vi "Page_AddProject.vi"(8 "error in (no error)":errorcluster, 11 "Configuration Paths in":T1) -> (0 "error out":errorcluster, 3 "Configuration Paths out":T1)   [LabVIEW 2010]
uses:
  Config cluster.ctl
panel:
  in  "Delete":bool
  in  "OK":bool
  in  "Selected Project Files":i32(listbox)
  in  "Configuration Files":i32(listbox)=-1
  in  "Cancel":bool
  in  "Add Proj":bool
  in  "Mode":enum16{"MIL", "HIL", "XiL"}(ring)
  # "1) Choose the type of test to be performed"
  # "2) Select the configuration files that will be used in the test(s)"
  # "Available Project Files"
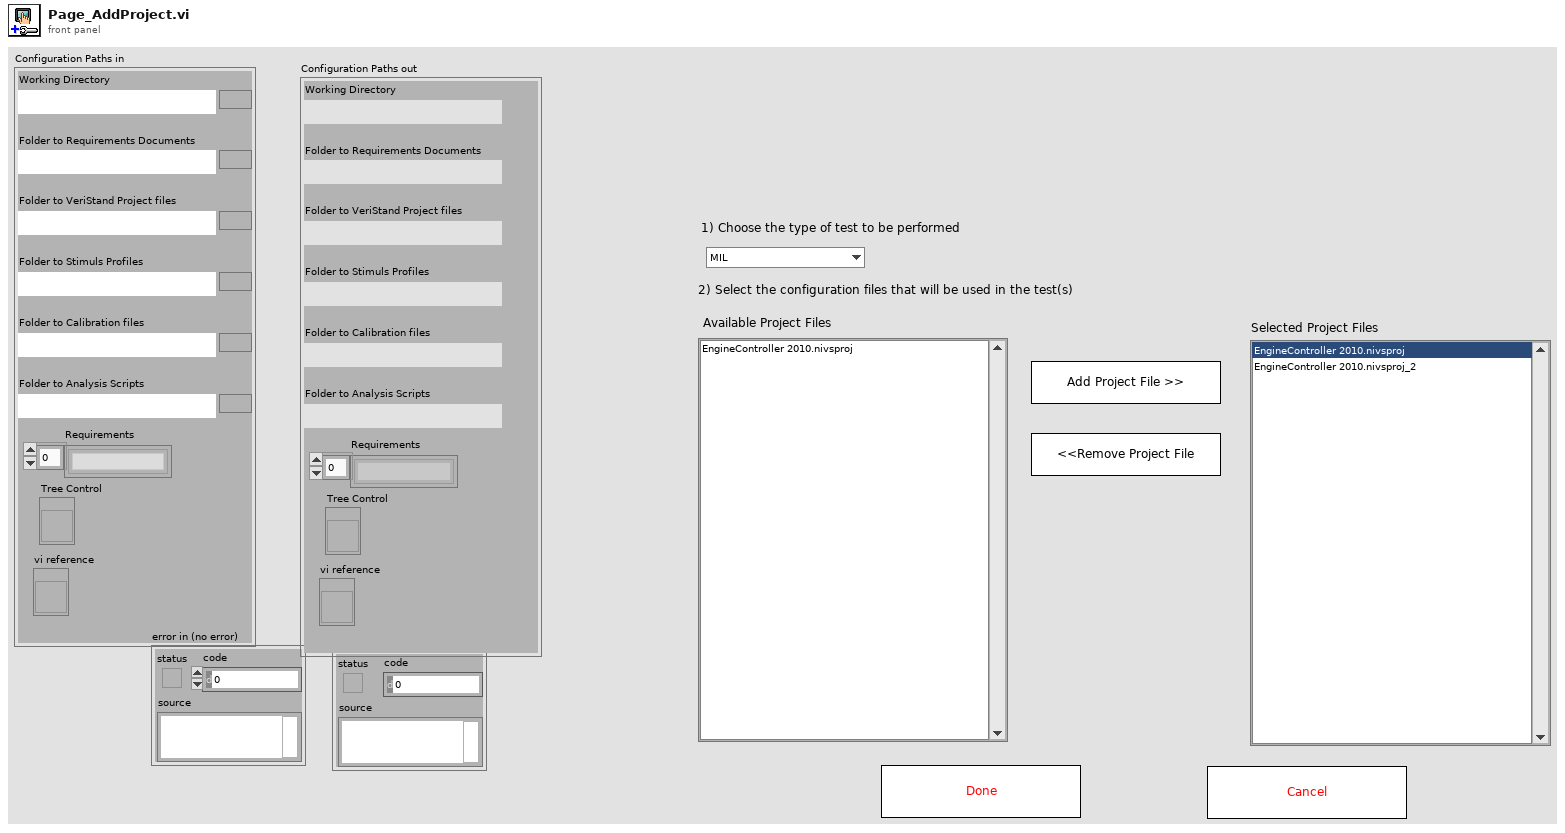
[diagram p1: front panel]
types:
  T1 = typedef "Config cluster.ctl" = cluster{"Working Directory":path, "Folder to Requirements Documents":path, "Folder to VeriStand Project files":path, "Folder to Stimuls Profiles":path, "Folder to Calibration files":path, "Folder to Analysis Scripts":path, "Requirements":string[], "Tree Control":refnum<vi>, "vi reference":refnum<vi>}
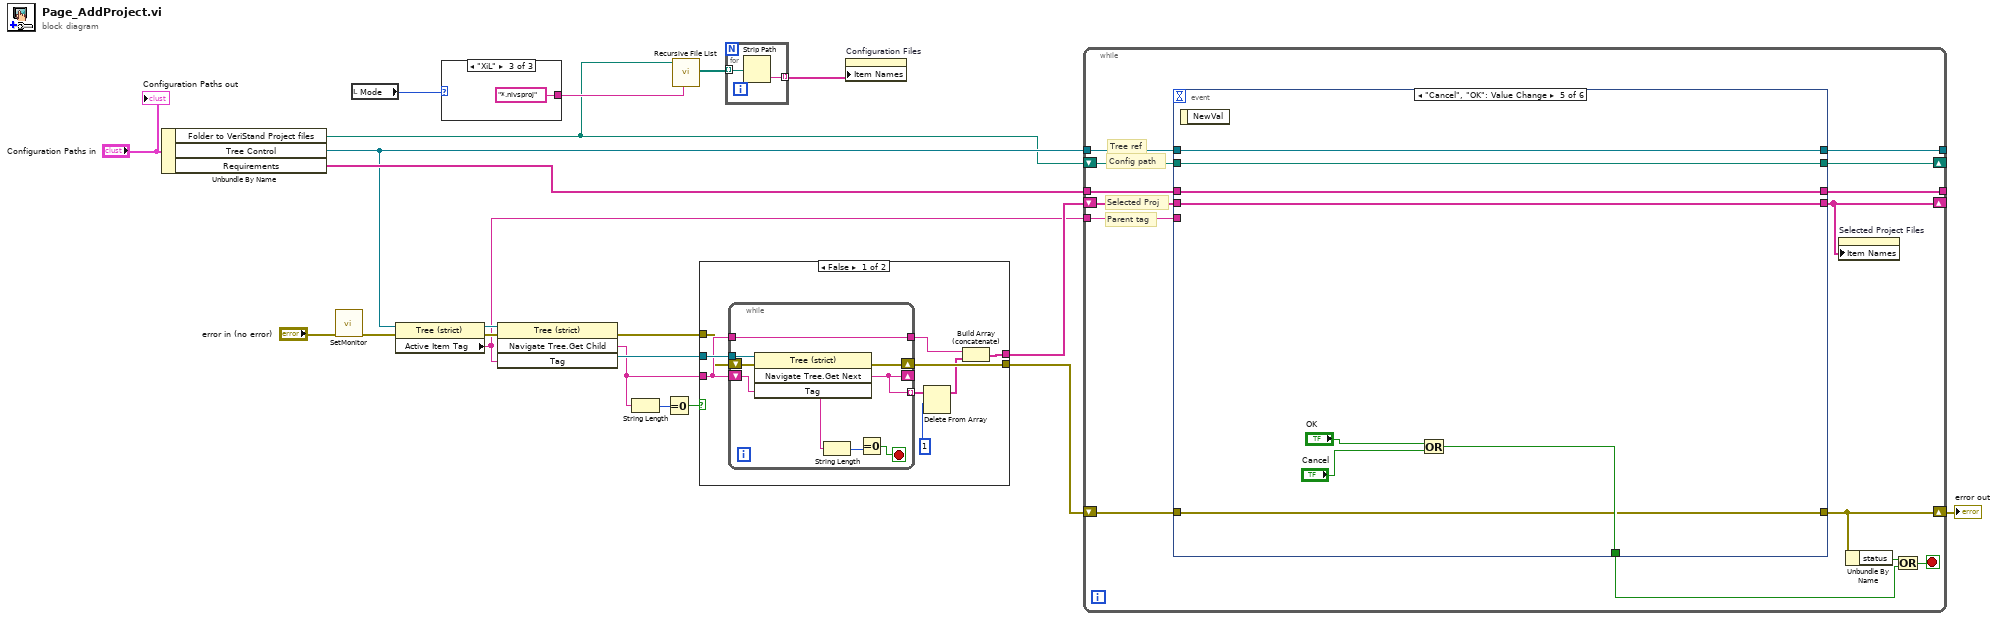
[diagram p0: block diagram]
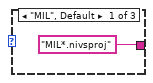
[diagram p2: hidden frame]
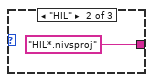
[diagram p3: hidden frame]
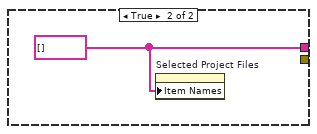
[diagram p4: hidden frame]
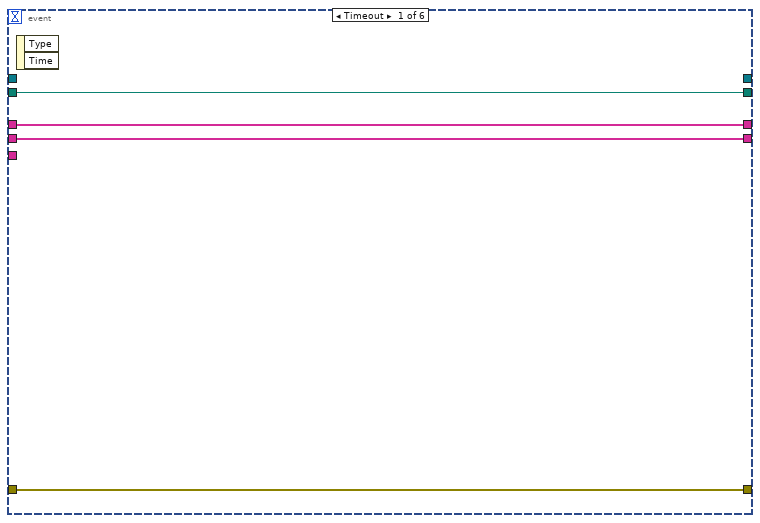
[diagram p5: hidden frame]
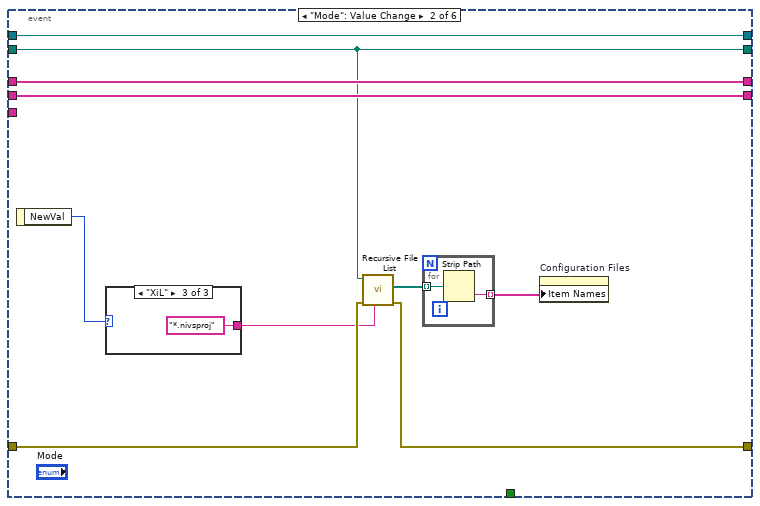
[diagram p6: hidden frame]
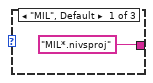
[diagram p7: hidden frame]
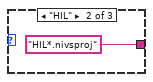
[diagram p8: hidden frame]
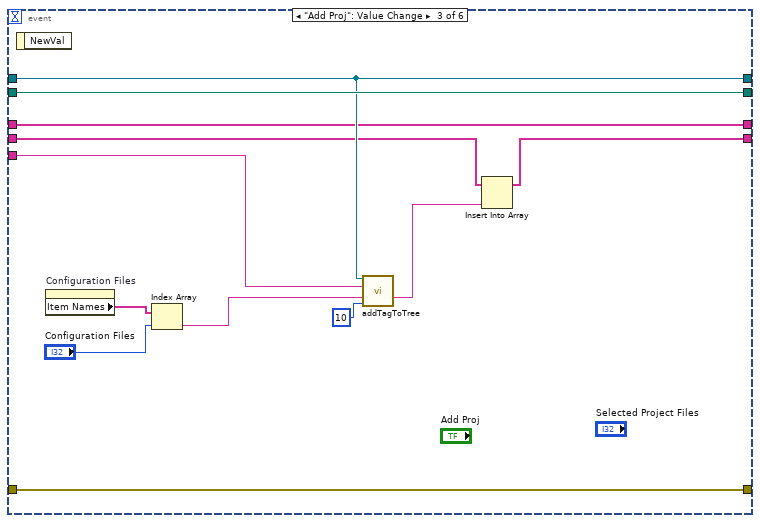
[diagram p9: hidden frame]
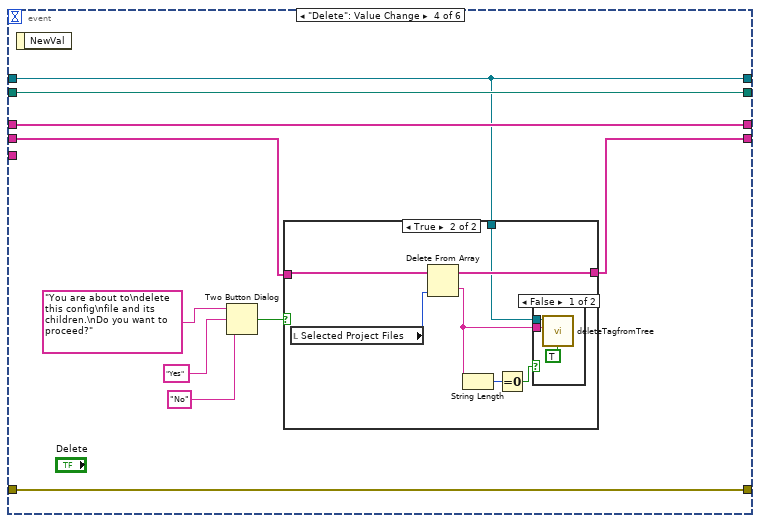
[diagram p10: hidden frame]
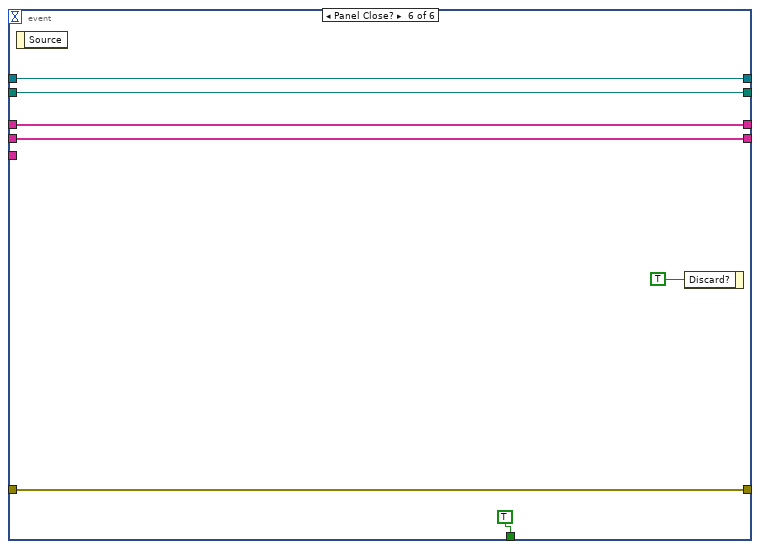
[diagram p13: hidden frame]
diagram:
  n1 = Unbundle By Name("Configuration Paths in") -> ("Folder to VeriStand Project files"=w3:path, "Tree Control"=w14:refnum<vi>, "Requirements"=w20:string[])
  n2 = call "SetMonitor.vi"("error in (no error)"="error in (no error)") -> ("error out"=w2:errorcluster)  [unwired: 9 in, 1 out]
  n3 = local read "Mode"() -> (w4:enum16{"MIL", "HIL", "XiL"})
  n4 = property class="Tree (strict)"(reference=w14, error in=w2) -> (reference out=w13:refnum<vi>, error out=w11:errorcluster, "Active Item Tag"=w8:string)
  n5 = case shown="\"XiL\"" w4 {
    tunnel: ["MIL*.nivsproj" ("name or relative path") "HIL*.nivsproj" ("name or relative path") "*.nivsproj" ("name or relative path")] -> w5
    frame "MIL", Default {
    }
    frame "HIL" {
    }
    frame "XiL" {
    }
  }
  n6 = invoke on="Invoke Node" class="Tree (strict)" method="Navigate Tree.Get Child"(reference=w13, error in=w11, "Tag"=w8) -> (reference out=w19:refnum<vi>, error out=w15:errorcluster, "Navigate Tree:Get Child"=w18:string)  [unwired: 1 in, 1 out]
  n7 = String Length(string=w18) -> (length=w17:i32)
  n8 = Equal To 0?(x=w17) -> (x = 0?=w16:bool)
  n9 = call <vilib>:"Recursive File List.vi"("pattern"=w5, "Folder Path"=w3) -> ("All Files in Dir"=w7:path[])  [unwired: 5 in, 4 out]
  n10 = case shown="False" w16 {
    tunnel: [w33 _] -> w10
    tunnel: w19 -> [w32 _]
    tunnel: [w28 w42] -> w12
    tunnel: w18 -> [w30 _]
    tunnel: w15 -> [w27 _]
    frame False {
      n11 = while {
        shift-right: [w38] -> _
        shift-left: w30 -> [w37]
        tunnel: [w38] -> w29 mode=indexing
        tunnel: w32 -> [w36]
        tunnel: [w35] -> w31
        tunnel: w30 -> [w35]
        shift-right: [w39] -> w33
        shift-left: w27 -> [w34]
        stop <- w40 stop-if-true
        n12 = invoke on="Invoke Node" class="Tree (strict)" method="Navigate Tree.Get Next"(reference=w36, error in=w34, "Tag"=w37) -> (error out=w39:errorcluster, "Navigate Tree:Get Next Item"=w38:string)  [unwired: 1 in, 2 out]
        n13 = String Length(string=w38) -> (length=w41:i32)
        n14 = Equal To 0?(x=w41) -> (x = 0?=w40:bool)
      }
      n15 = Delete From Array(array=w29, length=1) -> (array with subset deleted=w26:string[])  [unwired: 1 in, 1 out]
      n16 = Build Array (concatenate)(w31, w26) -> (w28:string[])
    }
    frame True {
      w42 = string[] []
      n17 = property on="Selected Project Files" class="LstBox (strict)"("Item Names"=w42) -> ()  [unwired: 2 in, 2 out]
    }
  }
  n18 = for {
    tunnel: w7 -> [w44] mode=indexing
    tunnel: [w43] -> w6 mode=indexing
    n19 = Strip Path(path=w44) -> (name=w43:string)  [unwired: 1 out]
  }
  n20 = property on="Configuration Files" class="LstBox (strict)"("Item Names"=w6) -> ()  [unwired: 2 in, 2 out]
  n21 = while {
    tunnel: w14 -> [w58]
    tunnel: w20 -> [w57]
    shift-right: [w56] -> _
    shift-left: w3 -> [w55]
    tunnel: [w54] -> _
    tunnel: [w52] -> _
    shift-right: [w49] -> w9
    shift-left: w10 -> [w50]
    tunnel: w8 -> [w45]
    shift-right: [w51] -> _
    shift-left: w12 -> [w53]
    stop <- w46 stop-if-true
    # "Parent tag"
    # "Selected Proj"
    # "Tree ref"
    # "Config path"
    n22 = event shown="[4] \"Cancel\", \"OK\": Value Change" {
      selector: _ -> [_ _ _ _ _ _]
      dyn-events: _ -> [_ _ _ _ _ _]
      timeout: _ -> [_ _ _ _ _ _]
      tunnel: [_ _ _ _ w115 TRUE] -> w47
      tunnel: [w62 w63 w87 w98 w111 w121] -> w56
      tunnel: w58 -> [_ w70 w86 w92 w110 w120]
      tunnel: w57 -> [w60 w67 w85 w94 w113 w123]
      tunnel: w55 -> [w62 w63 w87 w98 w111 w121]
      tunnel: [_ w70 w86 w92 w110 w120] -> w54
      tunnel: w53 -> [w59 w66 w84 w93 w112 w122]
      tunnel: [w59 w66 w83 w91 w112 w122] -> w51
      tunnel: [w60 w67 w85 w94 w113 w123] -> w52
      tunnel: w50 -> [w61 w69 w82 w89 w114 w124]
      tunnel: [w61 w68 w82 w89 w114 w124] -> w49
      tunnel: w45 -> [_ _ w81 _ _ _]
      event Timeout {
        n23 = event-data() -> ()  [unwired: 1 in, 2 out]
      }
      event "Mode": Value Change {
        n24 = event-data() -> ("NewVal"=w65:enum16{"MIL", "HIL", "XiL"})  [unwired: 1 in]
        n25 = case shown="\"XiL\"" w65 {
          tunnel: ["MIL*.nivsproj" ("name or relative path") "HIL*.nivsproj" ("name or relative path") "*.nivsproj" ("name or relative path")] -> w64
          frame "MIL", Default {
          }
          frame "HIL" {
          }
          frame "XiL" {
          }
        }
        n26 = call <vilib>:"Recursive File List.vi"("pattern"=w64, "error in (no error)"=w69, "Folder Path"=w63) -> ("error out"=w68:errorcluster, "All Files in Dir"=w72:path[])  [unwired: 4 in, 3 out]
        n27 = for {
          tunnel: w72 -> [w77] mode=indexing
          tunnel: [w76] -> w71 mode=indexing
          n28 = Strip Path(path=w77) -> (name=w76:string)  [unwired: 1 out]
        }
        n29 = property on="Configuration Files" class="LstBox (strict)"("Item Names"=w71) -> ()  [unwired: 2 in, 2 out]
      }
      event "Add Proj": Value Change {
        n30 = event-data() -> ()  [unwired: 1 in, 1 out]
        n31 = property on="Configuration Files" class="LstBox (strict)"() -> ("Item Names"=w80:string[])  [unwired: 2 in, 2 out]
        n32 = Index Array(array=w80, index="Configuration Files") -> (element=w78:string)
        n33 = call "addTagToTree.vi"("Tree ref"=w86, "parent tag"=w81, "new tag"=w78, "Symbol"=10) -> ()  [unwired: 11 in, 1 out]
        n34 = Insert Into Array(array=w84, new element=w78) -> (w83:string[])  [unwired: 1 in]
      }
      event "Delete": Value Change {
        n35 = event-data() -> ()  [unwired: 1 in, 1 out]
        n36 = Two Button Dialog(message="You are about to\ndelete this config\nfile and its children.\nDo you want to proceed?", 1:"No" ("F button name (\"Cancel\")"), 2:"Yes" ("T button name (\"OK\")")) -> (T button?=w97:bool)
        n37 = case shown="True" w97 {
          tunnel: w93 -> [w99 w106]
          tunnel: [w99 w105] -> w91
          tunnel: w92 -> [_ w104]
          frame False {
          }
          frame True {
            n38 = local read "Selected Project Files"() -> (w103:i32)
            n39 = Delete From Array(array=w106, index=w103) -> (deleted portion=w102:string, array with subset deleted=w105:string[])  [unwired: 1 in]
            n40 = String Length(string=w102) -> (length=w101:i32)
            n41 = Equal To 0?(x=w101) -> (x = 0?=w100:bool)
            n42 = case shown="False" w100 {
              tunnel: w104 -> [w109 _]
              tunnel: w102 -> [w107 _]
              frame False {
                n43 = call "deleteTagfromTree.vi"("Delete Children?"=TRUE, "Tag"=w107, "Tree Ref"=w109) -> ()  [unwired: 7 in, 2 out]
              }
              frame True {
              }
            }
          }
        }
      }
      event "Cancel", "OK": Value Change {
        n44 = event-data() -> ()  [unwired: 1 in, 1 out]
        n45 = Or(x="OK", y="Cancel") -> (x .or. y?=w115:bool)
      }
      event Panel Close? {
        n46 = event-data() -> ()  [unwired: 1 in, 1 out]
        n47 = event-data("Discard?"=TRUE) -> ()  [unwired: 1 in, 1 out]
      }
    }
    n48 = property on="Selected Project Files" class="LstBox (strict)"("Item Names"=w51) -> ()  [unwired: 2 in, 2 out]
    n49 = Unbundle By Name(w49) -> ("status"=w48:bool)
    n50 = Or(x=w48, y=w47) -> (x .or. y?=w46:bool)
  }
  "error out" <- w9
  "Configuration Paths out" <- "Configuration Paths in"
